vi "Surface defect identify process.vi"(8 "error in (no error)":errorcluster, 11 "Fiber Auto Collimation state data in":refnum<class "Fiber Auto Collimation state data.lvclass">) -> (0 "error out":errorcluster, 3 "Fiber Auto Collimation state data out":refnum<class "Fiber Auto Collimation state data.lvclass">)   [LabVIEW 2018]
uses:
  State data/Fiber Auto Collimation state data.lvclass
  <userlib>/nLight Tidbits/Logging/Controls/Logging type choice.ctl
  State data/Fiber Auto Collimation state data.lvclass/Fiber Auto Collimation state data.ctl
  State data/Add Changed data.vi
  <instrlib>/nLight Instruments/Beam Profiler/Beam Profiler.lvclass
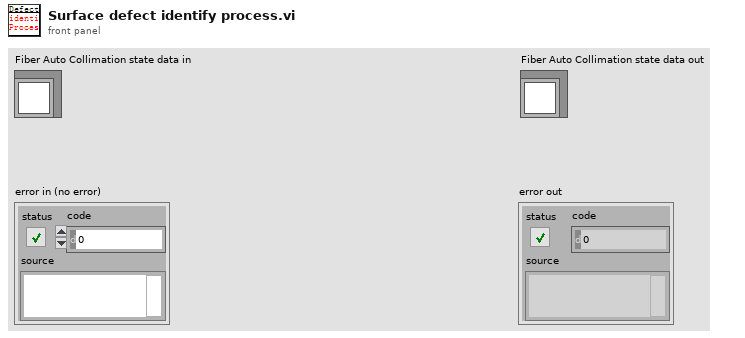
[diagram p1: front panel]
types:
  T1 = typedef "Logging type choice.ctl" = enum16{"No log type selected", "Testing start/stop", "Test progress", "Station startup/shutdown", "Station config change", "Recipe load/change", "Inventory transaction", "Instrument", "Debug"}
  T2 = typedef "Fiber Auto Collimation state data.lvclass/BV Data.ctl" = cluster{"Centroid X[um]":sgl, "Centroid Y[um]":sgl, "PeakResp.[%]":dbl, "Knife Edge X[mm]":sgl, "Knife Edge Y[mm]":sgl, "Circularity":sgl, "Collimation Result":bool}
  T3 = typedef "Test Parameters.ctl" = cluster{"Start position":dbl, "Peak Resp_min":dbl, "Circularity_min":dbl, "Beam Size Target":dbl, "Beam Size Percentage ":dbl, "Collimation Steps Data Path":string, "Collimation Data Path":string, "Defect detection Image Path":string, "Save Collimation Steps Data Enable":bool, "Defect detection Enable":bool, "Stop position":dbl}
  T4 = typedef "IMAQ Image.ctl" = refnum<image>
  T5 = typedef "VBAIInterface.ctl" = refnum<k21>
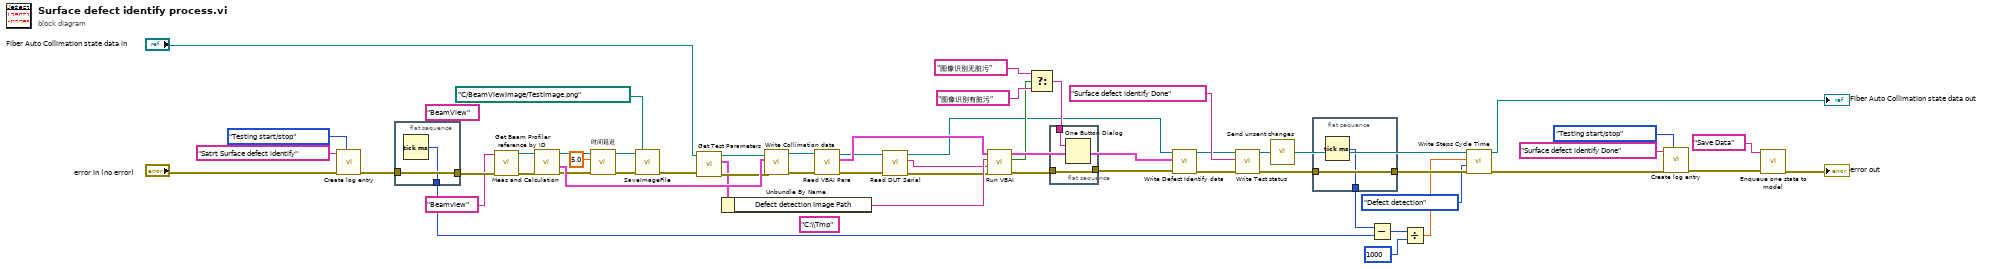
[diagram p0: block diagram]
diagram:
  (unwired) "C:\\Tmp" ("Path")
  (unwired) "BeamView"
  n1 = call <userlib>:"Create log entry.vi"("Logging type choice"=Logging_type_choice."Testing start/stop", "error in (no error)"="error in (no error)", "Brief log entry"="Satrt Surface defect identify") -> ("error out"=w30:errorcluster)  [unwired: 8 in]
  n2 = flat-sequence {
    tunnel: w30 -> [w57]
    tunnel: [w57] -> w29
    tunnel: [w56] -> w26
    frame #0 {
      n3 = Tick Count (ms)() -> (millisecond timer value=w56:u32)
    }
  }
  n4 = call <instrlib>:"Get Beam Profiler reference by ID.vi"("error in (no error)"=w29, "Identifier"="Beamview") -> ("error out"=w37:errorcluster, "Beam Profiler out"=w36:refnum<class "Beam Profiler.lvclass">)  [unwired: 8 in]
  n5 = call "Meas and Calculation.vi"("error in (no error)"=w37, "Beam Profiler in"=w36) -> ("error out"=w3:errorcluster, "BV Data"=w33:T2, "Beam Profiler out"=w6:refnum<class "Beam Profiler.lvclass">)  [unwired: 6 in, 1 out]
  n6 = call "时间延迟"("error in (no error)"=w3, "Delay Time (s)"=5.0) -> ("error out"=w4:errorcluster)  [unwired: 9 in]
  n7 = call-dynamic "SaveImageFile.vi"("Path"=path "C:/BeamViewImage/TestImage.png", "error in (no error)"=w4, "Beam Profiler in"=w6) -> ("error out"=w7:errorcluster)  [unwired: 7 in, 1 out]
  n8 = call "Get Test Parameters.vi"("error in (no error)"=w7, "Fiber Auto Collimation state data in"="Fiber Auto Collimation state data in") -> ("error out"=w17:errorcluster, "TestParameters"=w14:T3, "Fiber Auto Collimation state data out"=w15:refnum<class "Fiber Auto Collimation state data.lvclass">)  [unwired: 7 in]
  n9 = Unbundle By Name(w14) -> ("Defect detection Image Path"=w13:string)
  n10 = call "Write Collimation data.vi"("error in (no error)"=w17, "BV Data"=w33, "Fiber Auto Collimation state data in"=w15) -> ("error out"=w35:errorcluster, "Fiber Auto Collimation state data out"=w34:refnum<class "Fiber Auto Collimation state data.lvclass">)  [unwired: 7 in]
  n11 = call "Read VBAI Para.vi"("error in (no error)"=w35, "Fiber Auto Collimation state data in"=w34) -> ("error out"=w12:errorcluster, "VBAI"=w39:cluster{"New Image":T4, "VBAI Session Out":T5}, "Fiber Auto Collimation state data out"=w11:refnum<class "Fiber Auto Collimation state data.lvclass">)  [unwired: 7 in]
  n12 = call "Read DUT Serial.vi"("error in (no error)"=w12, "Fiber Auto Collimation state data in"=w11) -> ("error out"=w10:errorcluster, "DUT Serial"=w8:string, "Fiber Auto Collimation state data out"=w9:refnum<class "Fiber Auto Collimation state data.lvclass">)  [unwired: 7 in]
  n13 = call "Run VBAI.vi"("error in"=w10, "SN"=w8, "Path"=w13, "VBAI"=w39) -> ("error out"=w41:errorcluster, "Result"=w38:bool, "Defect identify data"=w40:cluster{"Image":T4, "Measure Report":string})  [unwired: 5 in]
  n14 = Select(t="图像识别无脏污", s=w38, f="图像识别有脏污") -> (s? t:f=w42:string)
  n15 = flat-sequence {
    tunnel: w41 -> [w59]
    tunnel: [w59] -> w45
    tunnel: w42 -> [w58]
    frame #0 {
      n16 = One Button Dialog(message=w58) -> ()  [unwired: 1 in, 1 out]
    }
  }
  n17 = call "Write Defect Identify data.vi"("error in (no error)"=w45, "Defect Identify data"=w40, "Fiber Auto Collimation state data in"=w9) -> ("error out"=w53:errorcluster, "Fiber Auto Collimation state data out"=w52:refnum<class "Fiber Auto Collimation state data.lvclass">)  [unwired: 7 in]
  n18 = call "Write Test status.vi"("error in (no error)"=w53, "Test status"="Surface defect identify Done", "Fiber Auto Collimation state data in"=w52) -> ("error out"=w28:errorcluster, "Fiber Auto Collimation state data out"=w55:refnum<class "Fiber Auto Collimation state data.lvclass">)  [unwired: 7 in]
  n19 = call "Send unsent changes.vi"("Fiber Auto Collimation state data in"=w55) -> ("Fiber Auto Collimation state data out"=w22:refnum<class "Fiber Auto Collimation state data.lvclass">)  [unwired: 1 in]
  n20 = flat-sequence {
    tunnel: w28 -> [w61]
    tunnel: [w61] -> w23
    tunnel: [w60] -> w27
    frame #0 {
      n21 = Tick Count (ms)() -> (millisecond timer value=w60:u32)
    }
  }
  n22 = Subtract(x=w27, y=w26) -> (x-y=w25:u32)
  n23 = Divide(x=w25, y=1000) -> (x/y=w19:dbl)
  n24 = call "Write Steps Cycle Time.vi"("error in (no error)"=w23, "Steps Action"=enum16{"Collimation", "Defect detection"}."Defect detection", "Cycle Time"=w19, "Fiber Auto Collimation state data in"=w22) -> ("error out"=w21:errorcluster, "Fiber Auto Collimation state data out"=→"Fiber Auto Collimation state data out":refnum<class "Fiber Auto Collimation state data.lvclass">)  [unwired: 6 in]
  n25 = call <userlib>:"Create log entry.vi"("Logging type choice"=Logging_type_choice."Testing start/stop", "error in (no error)"=w21, "Brief log entry"="Surface defect identify Done") -> ("error out"=w46:errorcluster)  [unwired: 8 in]
  n26 = call "Enqueue one state to model.vi"("error in (no error)"=w46, "Enqueued state"="Save Data") -> ("error out"=→"error out":errorcluster)  [unwired: 9 in]
